vi "Teleop.vi"() -> ()   [LabVIEW 2016]
doc: "This VI is called for each TeleOp packet received from the DS where the robot is not disabled. It is often used to read from the joysticks and update I/O or to update setpoints for timed control loops. It should complete and return within 20 milliseconds or it may miss DS packets."
uses:
  <vilib>/Rock Robotics/WPI/Utilities/WPI_GetSetVariantRefNum.vi
  External/2ndContollerStatus.vi
  External/External.lvlib
panel:
  out "Angle1":u16
  out "Angle0":u16
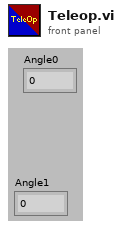
[diagram p1: front panel]
types:
  T1 = enum16{"A", "B", "X", "Y", "LB", "RB", "Back", "Start"}
  T2 = typedef "WPI_ServoDeviceRef.ctl" = cluster{"DeviceStatus":errorcluster, "PWM Channel":T3, "DeadBand":T4}
  T3 = typedef "FPGA_DIOPWMChannel.ctl" = enum8{"PWM 0", "PWM 1", "PWM 2", "PWM 3", "PWM 4", "PWM 5", "PWM 6", "PWM 7", "PWM 8", "PWM 9", "PWM MXP 0", "PWM MXP 1", "PWM MXP 2", "PWM MXP 3", "PWM MXP 4", "PWM MXP 5", "PWM MXP 6", "PWM MXP 7", "PWM MXP 8", "PWM MXP 9", "Invalid"}
  T4 = typedef "WPI_PWMDeadband.ctl" = cluster{"Name":string, "maxPositivePwm":i32, "minPositivePwm":i32, "centerPwm":i32, "maxNegativePwm":i32, "minNegativePwm":i32, "angularRange":u16}
  T5 = typedef "WPI_JoystickDevRef.ctl" = cluster{"Device":T6}
  T6 = typedef "WPI_JoystickDeviceEnum.ctl" = enum16{"USB 0", "USB 1", "USB 2", "USB 3", "USB 4", "USB 5"}
  T7 = typedef "WPI_RobotDriveDevRef.ctl" = cluster{"DevStatus":errorcluster, "Motors[]":T8[], "Square Inputs":bool, "Max Output":dbl}
  T8 = typedef "WPI_MotorControlDeviceRef.ctl" = cluster{"DeviceStatus":errorcluster, "Type":T9, "PWM":cluster{"PWM Channel":T3, "DeadBand":T4}, "CAN":cluster{"Device Number":u8, "SetOutput VI Ref":variant, "GetOutput VI Ref":variant, "Enable VI Ref":variant, "Disable VI Ref":variant, "Data":variant}, "Invert":bool}
  T9 = typedef "WPI_MotorControlType.ctl" = enum16{"PWM", "CAN"}
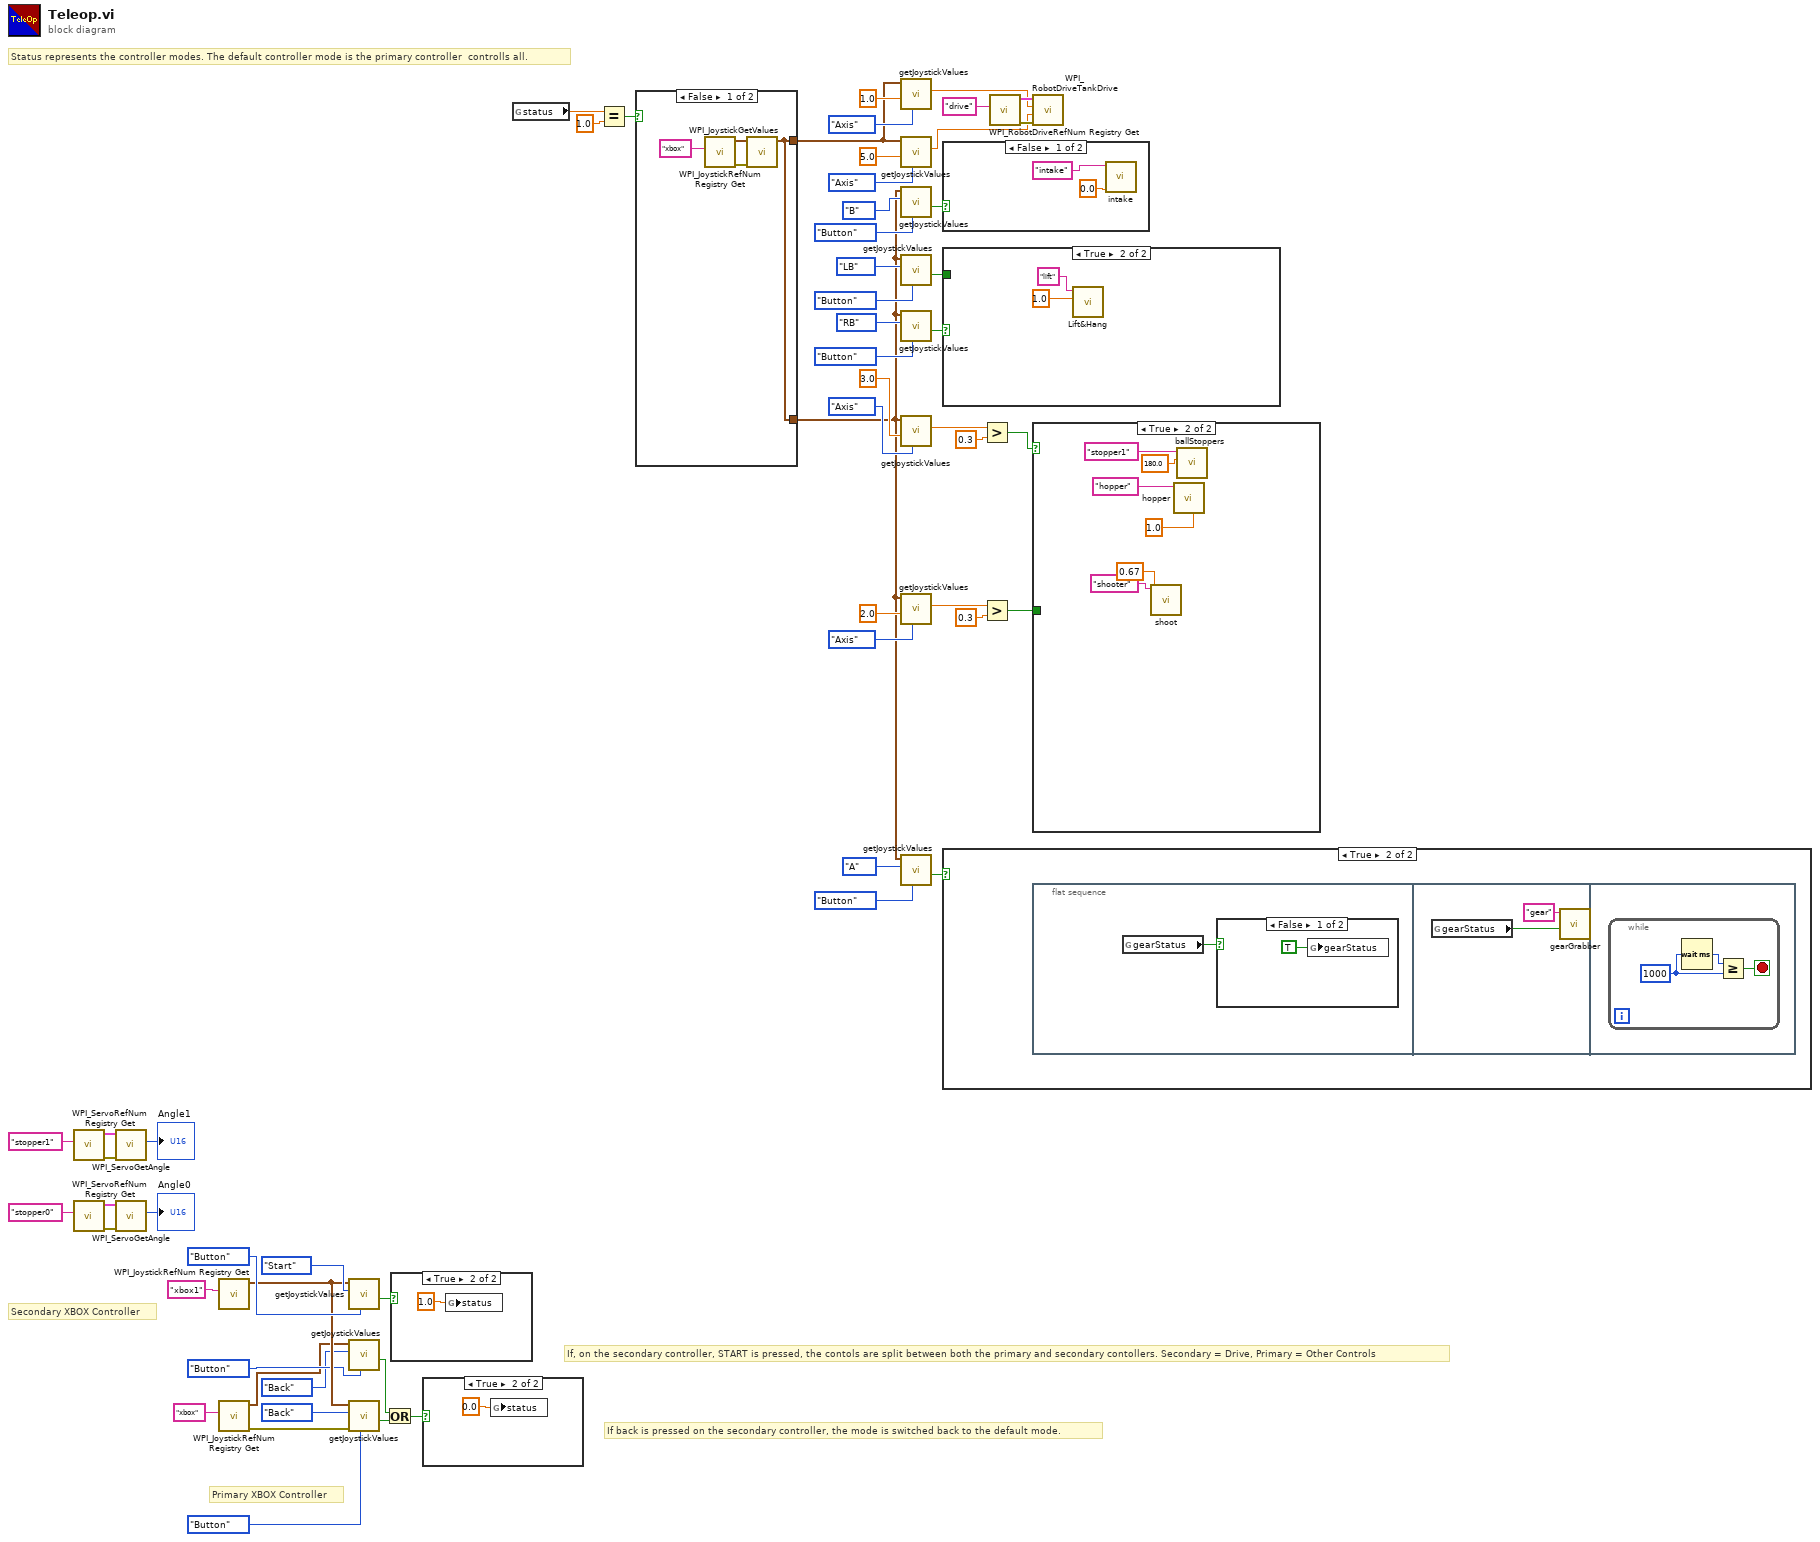
[diagram p0: block diagram]
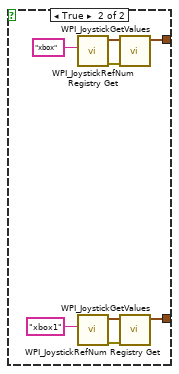
[diagram p2: hidden frame]
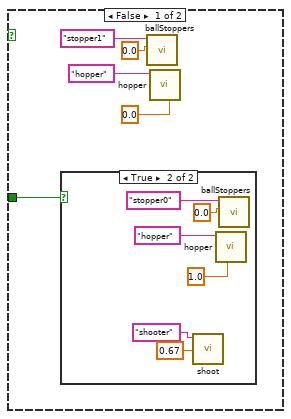
[diagram p3: hidden frame]
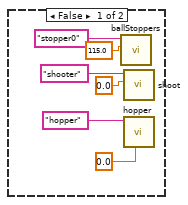
[diagram p4: hidden frame]
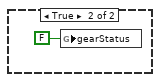
[diagram p6: hidden frame]
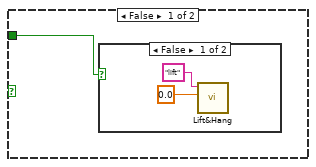
[diagram p7: hidden frame]
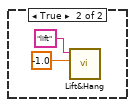
[diagram p8: hidden frame]
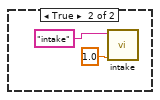
[diagram p9: hidden frame]
diagram:
  # "Status represents the controller modes. The default controller mode is the primary controller  controlls all."
  # "Secondary XBOX Controller"
  # "Primary XBOX Controller"
  # "If back is pressed on the secondary controller, the mode is switched back to the default mode."
  # "If, on the secondary controller, START is pressed, the contols are split between both the primary and secondary contollers. Secondary = Drive, Primary = Other Controls"
  n1 = call <vilib>:"WPI_ServoRefNum Registry Get.vi"("refnum name"="stopper1") -> ("error out"=w42:errorcluster, "ServoDeviceRef"=w41:T2)  [unwired: 9 in]
  n2 = call <vilib>:"WPI_ServoRefNum Registry Get.vi"("refnum name"="stopper0") -> ("error out"=w38:errorcluster, "ServoDeviceRef"=w37:T2)  [unwired: 9 in]
  n3 = call <vilib>:"WPI_ServoGetAngle.vi"("ServoDeviceRef"=w41, "error in (no error)"=w42) -> ("Angle"=→"Angle1":u16)  [unwired: 6 in, 2 out]
  n4 = call <vilib>:"WPI_ServoGetAngle.vi"("ServoDeviceRef"=w37, "error in (no error)"=w38) -> ("Angle"=→"Angle0":u16)  [unwired: 6 in, 2 out]
  n5 = call <vilib>:"WPI_JoystickRefNum Registry Get.vi"("refnum name"="xbox1" ("xbox1")) -> ("JoystickDevRef"=w54:T5)  [unwired: 9 in, 1 out]
  n6 = call <vilib>:"WPI_JoystickRefNum Registry Get.vi"("refnum name"="xbox" ("xbox")) -> ("error out"=w53:errorcluster, "JoystickDevRef"=w46:T5)  [unwired: 9 in]
  n7 = call "getJoystickValues.vi"("Mode"=enum16{"Axis", "Button"}."Button", "buttonType"=T1."Start", "JoystickDevRef"=w54) -> ("Button Pressed"=w49:bool)  [unwired: 5 in, 3 out]
  n8 = call "getJoystickValues.vi"("Mode"=enum16{"Axis", "Button"}."Button", "buttonType"=T1."Back", "JoystickDevRef"=w46) -> ("Button Pressed"=w47:bool)  [unwired: 5 in, 3 out]
  n9 = call "getJoystickValues.vi"("Mode"=enum16{"Axis", "Button"}."Button", "error in (no error)"=w53, "buttonType"=T1."Back", "JoystickDevRef"=w54) -> ("Button Pressed"=w48:bool)  [unwired: 4 in, 3 out]
  n10 = Or(x=w47, y=w48) -> (x .or. y?=w45:bool)
  n11 = case shown="True" w49 {
    frame False {
    }
    frame True {
      n12 = global write "2ndContollerStatus.vi" "status"(1.0 ("status")) -> ()
    }
  }
  n13 = case shown="True" w45 {
    frame False {
    }
    frame True {
      n14 = global write "2ndContollerStatus.vi" "status"(0.0 ("status")) -> ()
    }
  }
  n15 = global read "2ndContollerStatus.vi" "status"() -> (w11:dbl)
  n16 = Equal?(x=w11, y=1.0) -> (x = y?=w9:bool)
  n17 = case shown="False" w9 {
    tunnel: [w62 w70] -> w3
    tunnel: [w62 w66] -> w8
    frame False {
      n18 = call <vilib>:"WPI_JoystickRefNum Registry Get.vi"("refnum name"="xbox") -> ("error out"=w64:errorcluster, "JoystickDevRef"=w63:T5)  [unwired: 9 in]
      n19 = call <vilib>:"WPI_JoystickGetValues.vi"("error in (no error)"=w64, "JoystickDevRef"=w63) -> ("JoystickDevRef"=w62:T5)  [unwired: 5 in, 4 out]
    }
    frame True {
      n20 = call <vilib>:"WPI_JoystickRefNum Registry Get.vi"("refnum name"="xbox") -> ("error out"=w72:errorcluster, "JoystickDevRef"=w71:T5)  [unwired: 9 in]
      n21 = call <vilib>:"WPI_JoystickRefNum Registry Get.vi"("refnum name"="xbox1") -> ("error out"=w68:errorcluster, "JoystickDevRef"=w67:T5)  [unwired: 9 in]
      n22 = call <vilib>:"WPI_JoystickGetValues.vi"("error in (no error)"=w72, "JoystickDevRef"=w71) -> ("JoystickDevRef"=w70:T5)  [unwired: 5 in, 4 out]
      n23 = call <vilib>:"WPI_JoystickGetValues.vi"("error in (no error)"=w68, "JoystickDevRef"=w67) -> ("JoystickDevRef"=w66:T5)  [unwired: 5 in, 4 out]
    }
  }
  n24 = call "getJoystickValues.vi"("Mode"=enum16{"Axis", "Button"}."Axis", "Axis"=1.0, "JoystickDevRef"=w3) -> ("Value"=w5:dbl)  [unwired: 5 in, 3 out]
  n25 = call "getJoystickValues.vi"("Mode"=enum16{"Axis", "Button"}."Axis", "Axis"=5.0, "JoystickDevRef"=w3) -> ("Value"=w4:dbl)  [unwired: 5 in, 3 out]
  n26 = call "getJoystickValues.vi"("Mode"=enum16{"Axis", "Button"}."Button", "buttonType"=T1."B", "JoystickDevRef"=w8) -> ("Button Pressed"=w36:bool)  [unwired: 5 in, 3 out]
  n27 = call "getJoystickValues.vi"("Mode"=enum16{"Axis", "Button"}."Button", "buttonType"=T1."LB", "JoystickDevRef"=w8) -> ("Button Pressed"=w26:bool)  [unwired: 5 in, 3 out]
  n28 = call "getJoystickValues.vi"("Mode"=enum16{"Axis", "Button"}."Button", "buttonType"=T1."RB", "JoystickDevRef"=w8) -> ("Button Pressed"=w31:bool)  [unwired: 5 in, 3 out]
  n29 = call "getJoystickValues.vi"("Mode"=enum16{"Axis", "Button"}."Axis", "Axis"=3.0, "JoystickDevRef"=w8) -> ("Value"=w13:dbl)  [unwired: 5 in, 3 out]
  n30 = call "getJoystickValues.vi"("Mode"=enum16{"Axis", "Button"}."Axis", "Axis"=2.0, "JoystickDevRef"=w8) -> ("Value"=w12:dbl)  [unwired: 5 in, 3 out]
  n31 = call "getJoystickValues.vi"("Mode"=enum16{"Axis", "Button"}."Button", "buttonType"=T1."A", "JoystickDevRef"=w8) -> ("Button Pressed"=w22:bool)  [unwired: 5 in, 3 out]
  n32 = case shown="False" w36 {
    frame False {
      n33 = call "intake.vi"("intakeSpeed"=0.0, "intake"="intake") -> ()  [unwired: 9 in, 1 out]
    }
    frame True {
      n34 = call "intake.vi"("intakeSpeed"=1.0, "intake"="intake") -> ()  [unwired: 9 in, 1 out]
    }
  }
  n35 = case shown="True" w31 {
    tunnel: w26 -> [w78 _]
    frame False {
      n36 = case shown="False" w78 {
        frame False {
          n37 = call "Lift&Hang.vi"("status"=0.0, "refnum name"="lift" ("lift")) -> ()  [unwired: 9 in, 1 out]
        }
        frame True {
          n38 = call "Lift&Hang.vi"("status"=-1.0, "refnum name"="lift" ("lift")) -> ()  [unwired: 9 in, 1 out]
        }
      }
    }
    frame True {
      n39 = call "Lift&Hang.vi"("status"=1.0, "refnum name"="lift" ("lift")) -> ()  [unwired: 9 in, 1 out]
    }
  }
  n40 = case shown="True" w22 {
    frame False {
    }
    frame True {
      n41 = flat-sequence {
        frame #0 {
          n42 = global read "2ndContollerStatus.vi" "gearStatus"() -> (w85:bool)
          n43 = case shown="False" w85 {
            frame False {
              n44 = global write "2ndContollerStatus.vi" "gearStatus"(TRUE ("gearStatus")) -> ()
            }
            frame True {
              n45 = global write "2ndContollerStatus.vi" "gearStatus"(FALSE ("gearStatus")) -> ()
            }
          }
        }
        frame #1 {
          n46 = global read "2ndContollerStatus.vi" "gearStatus"() -> (w88:bool)
          n47 = call "gearGrabber.vi"("gearStatus"=w88, "gear"="gear") -> ()  [unwired: 9 in, 1 out]
        }
        frame #2 {
          n48 = while {
            stop <- w92 stop-if-true
            w90 = u32 1000 ("milliseconds to wait")
            n49 = Wait (ms)(milliseconds to wait=w90) -> (millisecond timer value=w91:u32)
            n50 = Greater Or Equal?(x=w91, y=w90) -> (x >= y?=w92:bool)
          }
        }
      }
    }
  }
  n51 = Greater?(x=w13, y=0.3) -> (0:w15:bool)
  n52 = Greater?(x=w12, y=0.3) -> (0:w14:bool)
  n53 = call <vilib>:"WPI_RobotDriveRefNum Registry Get.vi"("refnum name"="drive") -> ("error out"=w24:errorcluster, "RobotDriveDevRef"=w25:T7)  [unwired: 9 in]
  n54 = call <vilib>:"WPI_RobotDriveTankDrive.vi"("error in (no error)"=w24, "Right axis value"=w4, "Left axis value"=w5, "RobotDriveDevRef"=w25) -> ()  [unwired: 5 in, 3 out]
  n55 = case shown="True" w15 {
    tunnel: w14 -> [w97 _]
    frame False {
      n56 = case shown="True" w97 {
        frame False {
          n57 = call "ballStoppers.vi"("stopperValue"=115.0, "stopper1 or stopper0"="stopper0") -> ()  [unwired: 9 in, 1 out]
          n58 = call "shoot.vi"("Motor Power"=0.0, "refnum name"="shooter") -> ()  [unwired: 9 in, 1 out]
          n59 = call "hopper.vi"("Left axis value"=0.0 ("Right axis value"), "hopper"="hopper") -> ()  [unwired: 9 in, 1 out]
        }
        frame True {
          n60 = call "shoot.vi"("Motor Power"=0.67, "refnum name"="shooter") -> ()  [unwired: 9 in, 1 out]
          n61 = call "hopper.vi"("Left axis value"=1.0, "hopper"="hopper") -> ()  [unwired: 9 in, 1 out]
          n62 = call "ballStoppers.vi"("stopperValue"=0.0, "stopper1 or stopper0"="stopper0") -> ()  [unwired: 9 in, 1 out]
        }
      }
      n63 = call "ballStoppers.vi"("stopperValue"=0.0, "stopper1 or stopper0"="stopper1") -> ()  [unwired: 9 in, 1 out]
      n64 = call "hopper.vi"("Right axis value"=0.0, "hopper"="hopper") -> ()  [unwired: 9 in, 1 out]
    }
    frame True {
      n65 = call "shoot.vi"("Motor Power"=0.67, "refnum name"="shooter") -> ()  [unwired: 9 in, 1 out]
      n66 = call "hopper.vi"("Right axis value"=1.0, "hopper"="hopper") -> ()  [unwired: 9 in, 1 out]
      n67 = call "ballStoppers.vi"("stopperValue"=180.0, "stopper1 or stopper0"="stopper1") -> ()  [unwired: 9 in, 1 out]
    }
  }
